vi "TUNA parse comms string.vi"(0 "Nav String":string="$,A,43,13,230,B,10,20,120,C,10,10,330,D,14,36,110,T,08,12,234\r") -> (1 "Command Mode":i32, 2 "command string":string, 3 "Valid?":bool)   [LabVIEW 2014]
doc: "This VI will parse the Tug navigation string for the Tug letters, A for example, and the time, T. It returns a cluster with the Tug / Time and three values as decimals."
panel:
  out "Header":string="T"
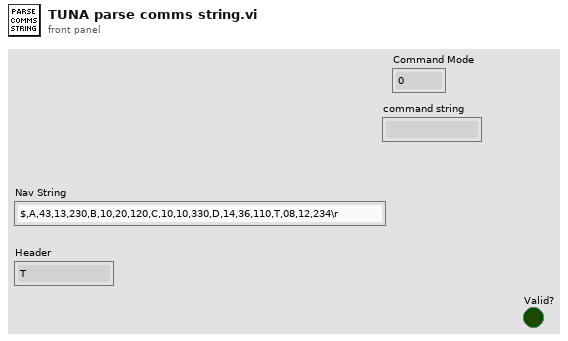
[diagram p1: front panel]
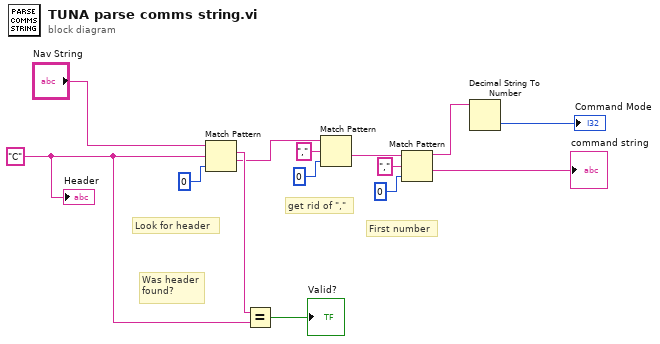
[diagram p0: block diagram]
diagram:
  w10 = "C" ("Header")
  # "First number"
  # "get rid of \",\""
  # "Was header\nfound?"
  # "Look for header"
  n1 = Match Pattern(string="Nav String", regular expression=w10, offset (0)=0) -> (match substring=w12:string, after substring=w3:string)  [unwired: 2 out]
  n2 = Equal?(x=w12, y=w10) -> (x = y?=→"Valid?":bool)
  n3 = Match Pattern(string=w3, regular expression=",", offset (0)=0) -> (after substring=w4:string)  [unwired: 3 out]
  n4 = Match Pattern(string=w4, regular expression=",", offset (0)=0) -> (before substring=w7:string, after substring=→"command string":string)  [unwired: 2 out]
  n5 = Decimal String To Number(string=w7) -> (number=→"Command Mode":i32)  [unwired: 2 in, 1 out]
  "Header" <- w10
